vi "Start.vi"(8 "Error In":errorcluster, 11 "IScope in":refnum<class "IScope.lvclass">) -> (0 "Error Out":errorcluster, 3 "IScope out":refnum<class "IScope.lvclass">)   [LabVIEW 2023, in "IScope.lvclass"]
uses:
  IScope.lvclass
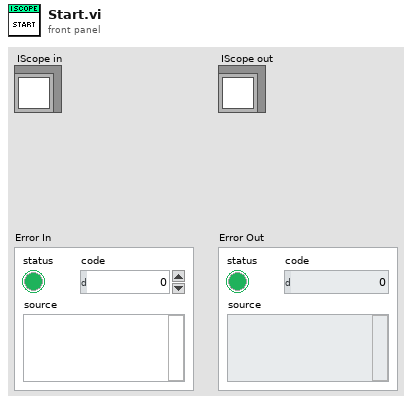
[diagram p1: front panel]
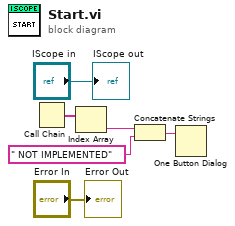
[diagram p0: block diagram]
diagram:
  n1 = Call Chain() -> (call chain=w4:string[])
  n2 = Index Array(array=w4) -> (element=w2:string)  [unwired: 1 in]
  n3 = Concatenate Strings(w2, " NOT IMPLEMENTED" ("string")) -> (w3:string)
  n4 = One Button Dialog(message=w3) -> ()  [unwired: 1 in, 1 out]
  "Error Out" <- "Error In"
  "IScope out" <- "IScope in"
